vi "LDA ReadEigenVectorsSize.vi"(8 "error in":errorcluster, 11 "LDA":refnum<class "LDA.lvclass">) -> (0 "error out":errorcluster, 1 "Cols":i32, 2 "Rows":i32, 3 "LDA":refnum<class "LDA.lvclass">)   [LabVIEW 2020, in "OpenLvVision_OpenCv.lvlib" / "LDA.lvclass"]
uses:
  LDA.lvclass
  C:/Users/lukas/Downloads/OpenLvVision_OpenCv/SourceCode/LabView/OpenLvVision_OpenCv/_LvHelpers/EdvrObject/EdvrObject.lvclass
  _LvHelpers/EdvrObject/EdvrObject.lvclass/EdvrObject.ctl
  OpenLvVision_OpenCv.lvlib
  _LvHelpers/EdvrObject/EdvrObject.lvclass
  Dlls/OlvOpenCvWrapper.dll
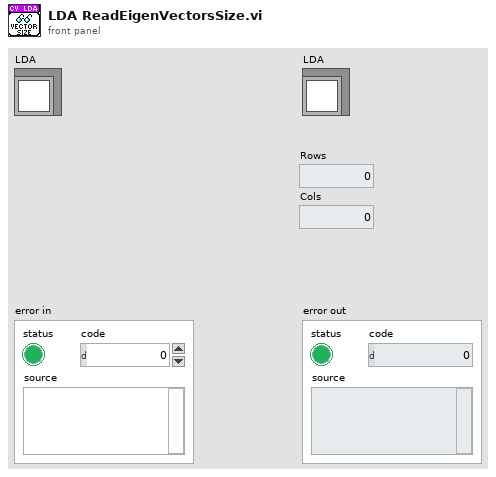
[diagram p1: front panel]
types:
  T1 = typedef "OpenLvVision_OpenCv.lvlib/EdvrObject.lvclass/Edvr.ctl" = refnum<data-value>
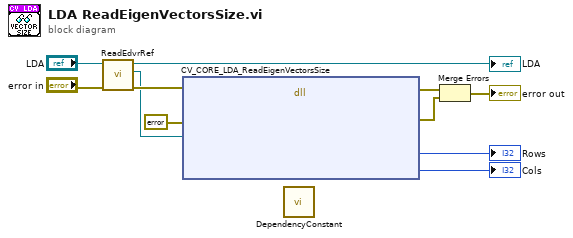
[diagram p0: block diagram]
diagram:
  n1 = call "ReadEdvrRef.vi"("error in (no error)"="error in", "EdvrObject in"="LDA") -> ("error out"=w2:errorcluster, "Edvr"=w1:T1, "EdvrObject out"=→"LDA":refnum<class "LDA.lvclass">)  [unwired: 7 in]
  n2 = dll-call lib="C:/Users/lukas/Downloads/OpenLvVision_OpenCv/SourceCode/LabView/OpenLvVision_OpenCv/Dlls/OlvOpenCvWrapper.dll" fn="CV_CORE_LDA_ReadEigenVectorsSize"(error in=w2, "Error"=errorcluster {"status"=FALSE, "code"=0, "source"=""} ("error out"), "edvrRef"=w1) -> (error out=w4:errorcluster, "Error"=w3:errorcluster, "Rows"=→"Rows":i32, "Cols"=→"Cols":i32)  [unwired: 6 in, 1 out]
  n3 = call "DependencyConstant.vi"() -> ()  [unwired: 12 in]
  n4 = Merge Errors(w4, w3) -> (→"error out":errorcluster)
